vi "Find Marker Location.vi"(2 "Marker Length":i32, 3 "Datastream Buffer":u8[](array[numeric])) -> (0 "Marker Appeared at":i32, 1 "Marker Appeared ?":bool)   [LabVIEW 2020, in "AoC 2022.lvlib"]
uses:
  AoC 2022.lvlib
  2ac3cfda-2155-437b-9cc3-3f96bb7126fc.vi
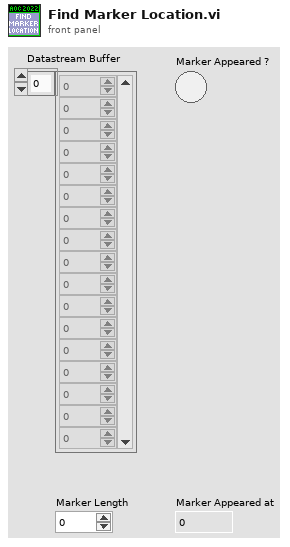
[diagram p1: front panel]
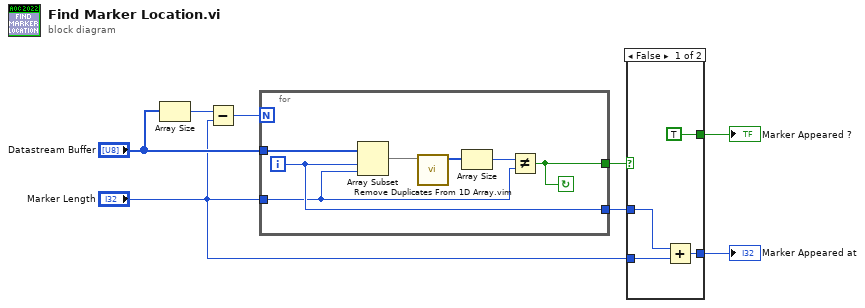
[diagram p0: block diagram]
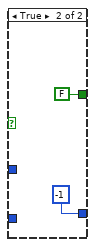
[diagram p2: hidden frame]
diagram:
  n1 = Array Size(array="Datastream Buffer") -> (size(s)=w8:i32)
  n2 = Subtract(x=w8, y="Marker Length") -> (x-y=w6:i32)
  n3 = for {
    N: w6 -> [_]
    tunnel: "Datastream Buffer" -> [w15]
    tunnel: "Marker Length" -> [w9]
    tunnel: [w12] -> w5
    tunnel: [w11] -> w2
    i -> [w12]
    stop <- w11 continue-if-true
    n4 = Array Subset(array=w15, index=w12, length=w9) -> (w14:u8[])
    n5 = call "Remove Duplicates From 1D Array.vim"("array"=w14) -> ("array with duplicates removed"=w13:u8[])  [unwired: 10 in]
    n6 = Array Size(array=w13) -> (size(s)=w10:i32)
    n7 = Not Equal?(x=w10, y=w9) -> (x != y?=w11:bool)
  }
  n8 = case shown="False" w2 {
    tunnel: w5 -> [w19 _]
    tunnel: "Marker Length" -> [w18 _]
    tunnel: [w17 -1] -> w3
    tunnel: [TRUE FALSE] -> w1
    frame False {
      n9 = Add(x=w19, y=w18) -> (x+y=w17:i32)
    }
    frame True {
    }
  }
  "Marker Appeared at" <- w3
  "Marker Appeared ?" <- w1
